vi "Send Run Config to all GDs.vi"(6 "Guardian ID or ALL":string, 7 "Button":T1, 8 "error in (no error)":errorcluster, 9 "Run Config Name":string, 10 "CSV Path":path, 11 "Guardian in":refnum<class "Guardian.lvclass">) -> (0 "error out":errorcluster, 3 "Guardian out":refnum<class "Guardian.lvclass">)   [LabVIEW 2026, in "TALOS.lvlib" / "Guardian.lvlib" / "Guardian.lvclass"]
doc: "This VI sends a message to all the other Guardians, by writing it on Broadcast_Guardian SV."
uses:
  Guardian.lvclass
  C:/LabVIEW Code/TALOS/builds/Actor Framework PPL/Actor Framework.lvlibp/1abvi3w/vi.lib/ActorFramework/Actor/Actor.lvclass
  Buttons_UI.ctl
  Guardian.lvclass/Guardian.ctl
  Guardian Messages/Message to Other Guardian Msg/Message to Other Guardian Msg.lvclass/Message to Other Guardian Msg.ctl
  Guardian Messages/TCP-SV Message Interpreter Msg/TCP-SV Message Interpreter Msg.lvclass/TCP-SV Message Interpreter Msg.ctl
  Ancestor/Ancestor/Ancestor.lvclass/Ancestor.ctl
  Support VIs/Generate Error.vi
  FGV/Error Memory/Get Error Description.vi
  Support VIs/Get PC name.vi
  Ancestor/Ancestor/Read ID.vi
  Support VIs/Get Class Name.vi
  <vilib>/Utility/error.llb/Clear Errors.vi
  FGV/Error Memory/Error Memory Core.vi
  <vilib>/AdvancedString/Delimited String to 1D String Array.vi
  <vilib>/AdvancedString/Delimited String to 1D String Array (string).vi
  Support VIs/Circus Root Path.vi
  FGV/Error Memory/Error Crt Lvl checker.vi
  FGV/Error Memory/Error Memory Core.vi/40c8088d-b597-4017-91af-faa98e00292e.vi
  FGV/Error Memory/Error Memory Core.vi/d4a3ab98-063c-4e44-b43d-fbdcfe6c2be2.vi
  Support VIs/Global Constants.vi
  builds/Actor Framework PPL/Actor Framework.lvlibp/1abvi3w/vi.lib/ActorFramework/Message Enqueuer/Enqueue.vi
  Support VIs/Global Memory.vi
  <vilib>/Utility/LVClass/Get LV Class Name.vi
  Support VIs/Is in Packed Library.vi
  Support VIs/TALOS Root path.vi
  <vilib>/Utility/error.llb/General Error Handler.vi
  Support VIs/Error Log.vi
  Guardian Messages/Message to Other Guardian Msg/Message to Other Guardian Msg.lvclass
  Guardian Messages/TCP-SV Message Interpreter Msg/TCP-SV Message Interpreter Msg.lvclass
  Ancestor/Ancestor/Ancestor.lvclass
  <vilib>/Comparison/Equal/Equal Functor/Equal Functor.lvclass
  Classes/Guardian List/Guardian List.lvclass
  builds/Actor Framework PPL/Actor Framework.lvlibp/1abvi3w/vi.lib/ActorFramework/Actor/Actor.lvclass
  TALOS.lvlib
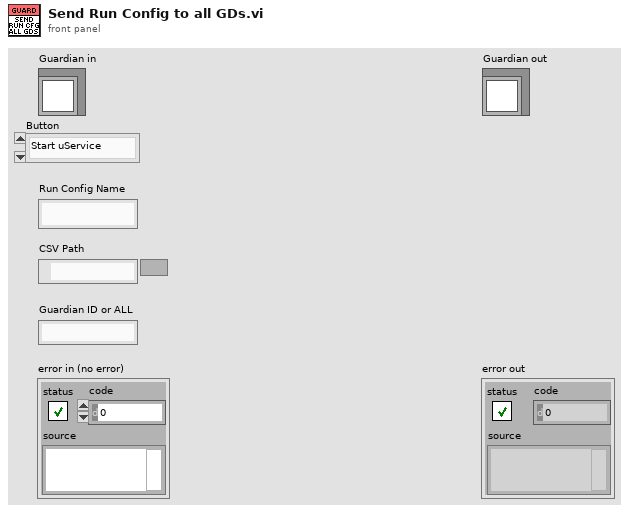
[diagram p1: front panel]
types:
  T1 = typedef "TALOS.lvlib/Guardian.lvlib/Guardian.lvclass/Buttons_UI.ctl" = enum16{"Start uService", "Kill uService", "Stop uService", "Stop", "Start online checks", "Stop online checks", "Send Pat to all GDs", "Reload INI files", "Update from GIT", "RUN", "Reset ABORT", "Check Bearer", "Send I Exist", "Change Run Config", "Add uSs from Config", "Realign uSs from Config", "Send Run Config to GD"}
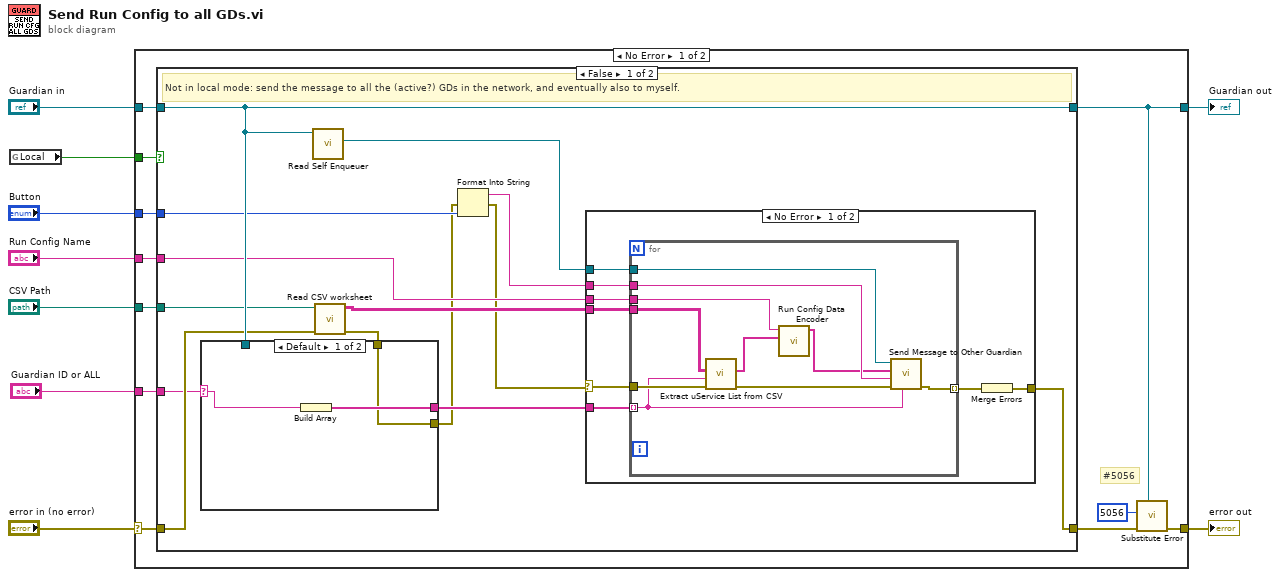
[diagram p0: block diagram]
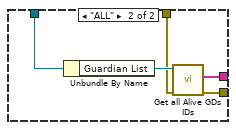
[diagram p2: hidden frame]
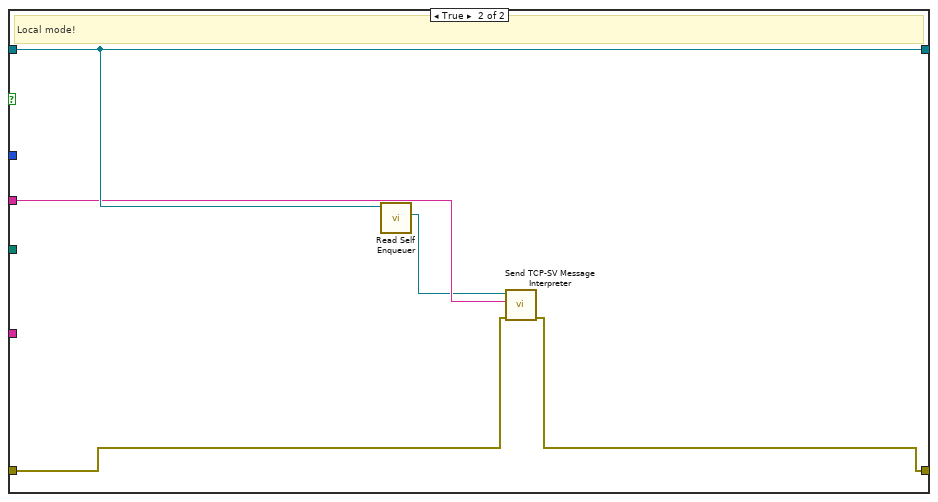
[diagram p4: hidden frame]
diagram:
  n1 = global read "Global Constants.vi" "Local"() -> (w4:bool)
  n2 = case shown="No Error" "error in (no error)" {
    selector: "error in (no error)" -> [w18 w68]
    tunnel: [w15 w68] -> w8
    tunnel: [w14 w67] -> w6
    tunnel: "Guardian in" -> [w19 w67]
    tunnel: "Run Config Name" -> [w20 _]
    tunnel: w4 -> [w17 _]
    tunnel: "Button" -> [w12 _]
    tunnel: "CSV Path" -> [w11 _]
    tunnel: "Guardian ID or ALL" -> [w10 _]
    frame No Error {
      # "#5056"
      n3 = case shown="False" w17 {
        tunnel: [w34 w65] -> w16
        tunnel: w20 -> [w26 w63]
        tunnel: w19 -> [w32 w64]
        tunnel: w18 -> [w29 w66]
        tunnel: [w32 w64] -> w14
        tunnel: w12 -> [w31 _]
        tunnel: w11 -> [w27 _]
        tunnel: w10 -> [w21 _]
        frame False {
          # "Not in local mode: send the message to all the (active?) GDs in the network, and eventually also to myself."
          n4 = call "Read Self Enqueuer.vi"("Actor"=w32) -> ("Self Enqueuer"=w33:refnum<class "Message Enqueuer.lvclass">)  [unwired: 10 in]
          n5 = call "Read CSV worksheet.vi"("error in (no error)"=w29, "appended path"=w27) -> ("error out"=w28:errorcluster, "Sheet"=w24:string[][])  [unwired: 8 in]
          n6 = case shown="Default" w21 {
            selector: w21 -> [w37 _]
            tunnel: w32 -> [_ w42]
            tunnel: w28 -> [w35 w40]
            tunnel: [w36 w39] -> w25
            tunnel: [w35 w38] -> w23
            frame Default {
              n7 = Build Array(w37) -> (w36:string[])
            }
            frame "ALL" {
              n8 = Unbundle By Name(w42) -> ("Guardian List"=w41:refnum<class "Guardian List.lvclass">)
              n9 = call-dynamic "Get all Alive GDs IDs.vi"("error in (no error)"=w40, "Guardian List in"=w41) -> ("error out"=w38:errorcluster, "Alive GDs IDs"=w39:string[])  [unwired: 7 in, 1 out]
            }
          }
          n10 = Format Into String(error in=w23, w31) -> (resulting string=w30:string, error out=w22:errorcluster)  [unwired: 2 in]
          n11 = case shown="No Error" w22 {
            selector: w22 -> [w47 w61]
            tunnel: [w50 w61] -> w34
            tunnel: w33 -> [w48 _]
            tunnel: w30 -> [w46 _]
            tunnel: w26 -> [w45 _]
            tunnel: w25 -> [w44 _]
            tunnel: w24 -> [w43 _]
            frame No Error {
              n12 = for {
                tunnel: [w59] -> w49 mode=indexing
                tunnel: w48 -> [w60]
                tunnel: w47 -> [w57]
                tunnel: w46 -> [w58]
                tunnel: w45 -> [w56]
                tunnel: w44 -> [w52] mode=indexing
                tunnel: w43 -> [w55]
                n13 = call "Extract uService List from CSV.vi"("error in (no error)"=w57, "Guardian ID"=w52, "CSV table"=w55) -> ("error out"=w53:errorcluster, "uS array"=w54:string[])  [unwired: 7 in]
                n14 = call "Run Config Data Encoder.vi"("uS array"=w54, "Run Config Name"=w56) -> ("Run config data array"=w51:string[])  [unwired: 9 in]
                n15 = call "Send Message to Other Guardian.vi"("Guardian ID"=w52, "error in (no error)"=w53, "Message"=w58, "Data"=w51, "Message Enqueuer"=w60) -> ("error out"=w59:errorcluster)  [unwired: 5 in, 1 out]
              }
              n16 = Merge Errors(w49) -> (w50:errorcluster)
            }
            frame Error {
            }
          }
        }
        frame True {
          # "Local mode!"
          n17 = call "Read Self Enqueuer.vi"("Actor"=w64) -> ("Self Enqueuer"=w62:refnum<class "Message Enqueuer.lvclass">)  [unwired: 10 in]
          n18 = call "Send TCP-SV Message Interpreter.vi"("error in (no error)"=w66, "Message"=w63, "Message Enqueuer"=w62) -> ("error out"=w65:errorcluster)  [unwired: 7 in, 1 out]
        }
      }
      n19 = call "Substitute Error.vi"("LabVIEW Object"=w14, "error in (no error)"=w16, "Error Code"=5056) -> ("error out"=w15:errorcluster)  [unwired: 8 in]
    }
    frame Error {
    }
  }
  "error out" <- w8
  "Guardian out" <- w6
